vi "SPECTRUM Set Settings_AM1.vi"(2 "error in (no error)":errorcluster, 3 "Cluster":T2 {"verticalUnit" items=["SpectrumVerticalUnit_dBm", "SpectrumVerticalUnit_Watt", "SpectrumVerticalUnit_Volt", "SpectrumVerticalUnit_Amp", "SpectrumVerticalUnit_dBmV"]; "window" items=["SpectrumWindow_Kaiser", "SpectrumWindow_Mil6dB", "SpectrumWindow_BlackmanHarris", "SpectrumWindow_Rectangle", "SpectrumWindow_FlatTop", "SpectrumWindow_Hann"]}) -> (0 "error out":errorcluster, 1 "function return":u32(ring))   [LabVIEW 2016]
doc: "RSA_API_DLL ReturnStatus SPECTRUM_SetSettings(Spectrum_Settings settings);"
uses:
  <userlib>/RSA_API/RSA_API.lvlib
  Tektronix/RSA_API/lib/x86/RSA_API.dll
panel:
  out "number":i32
  out "traceLength":T1(ring)
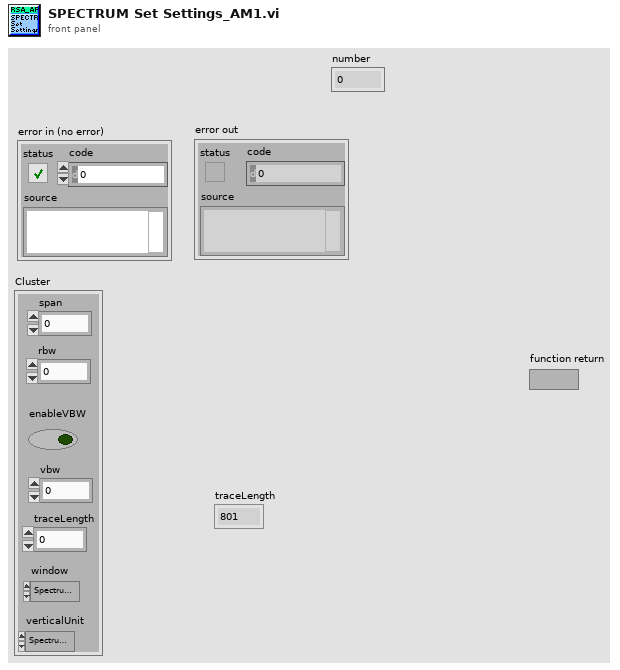
[diagram p1: front panel]
types:
  T1 = enum16{"801", "2401", "4001", "8001", "10401", "16001", "32001", "64001"}
  T2 = cluster{"span":dbl, "rbw":dbl, "enableVBW":bool, "vbw":dbl, "traceLength":dbl, "window":u32, "verticalUnit":u32}
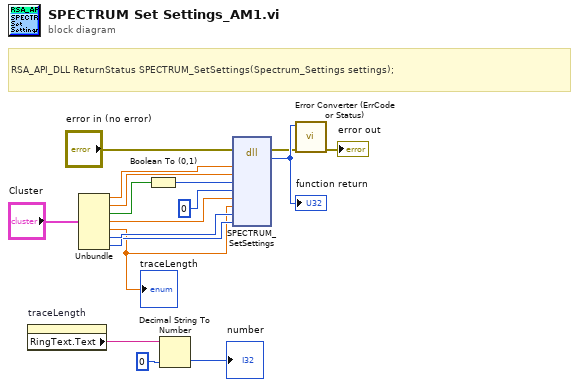
[diagram p0: block diagram]
diagram:
  # "RSA_API_DLL ReturnStatus SPECTRUM_SetSettings(Spectrum_Settings settings);"
  n1 = property on="traceLength" class="Enum (strict)"() -> ("RingText.Text"=w4:string)  [unwired: 2 in, 2 out]
  n2 = Unbundle("Cluster") -> ("span"=w12:dbl, "rbw"=w11:dbl, "enableVBW"=w10:bool, "vbw"=w9:dbl, "traceLength"=w1:dbl, "window"=w8:u32, "verticalUnit"=w7:u32)
  "traceLength" <- w1
  n3 = Boolean To (0,1)(Boolean=w10) -> (0, 1=w16:i16)
  n4 = Decimal String To Number(string=w4, default (0L)=0 ("default (0 I32)")) -> (number=→"number":i32)  [unwired: 1 in, 1 out]
  n5 = dll-call lib="C:/Tektronix/RSA_API/lib/x86/RSA_API.dll" fn="SPECTRUM_SetSettings"(error in="error in (no error)", "span"=w12, "rbw"=w11, "enableVBW"=w16, "@dummy control@"=i8 0, "vbw"=w9, "traceLength"=w1, "window"=w8, "verticalUnit"=w7) -> (error out=w15:errorcluster, "return type"=w17:u32)  [unwired: 10 in, 1 out]
  "function return" <- w17
  n6 = call <userlib>:"Error Converter (ErrCode or Status).vi"("error in (no error)"=w15, "error code"=w17) -> ("error out"=→"error out":errorcluster)  [unwired: 9 in]
